vi "open_plotter.vi"(10 "Break":refnum<vi>) -> ()   [LabVIEW 2019]
panel:
  out "Output File Loaded?":bool
  in  "Load Simulation":bool
  in  "Close":bool
  out "# Lines Plot":i32
  in  "Parameters to Plot":string(tree)="_3"
  out "Output Files Path":path caption="selected path"
  in  "Open Button":bool
  in  "Clear Plot Selection":bool
  in  "Plot":bool
  # "Biogas Plotter"
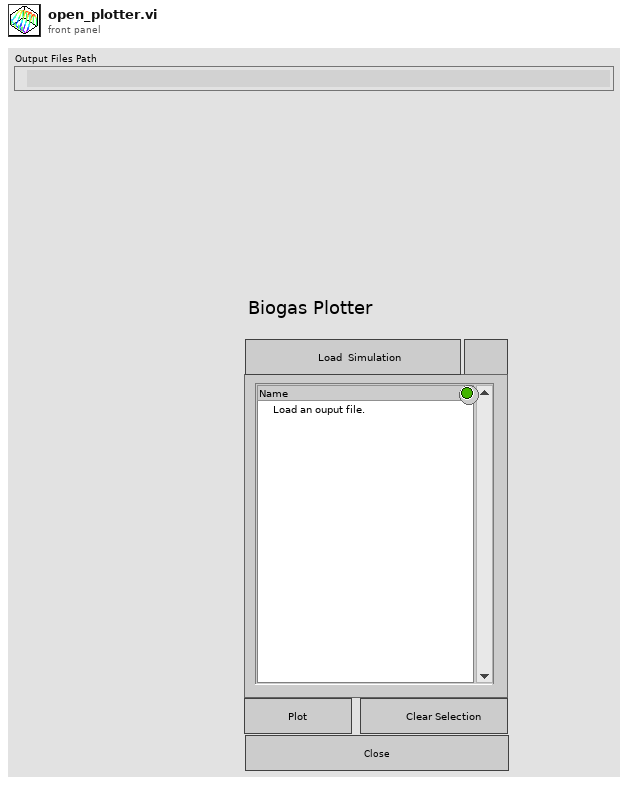
[diagram p1: front panel]
types:
  T1 = typedef "LVPoint32TypeDef.ctl" = cluster{"Horizontal":i32, "Vertical":i32}
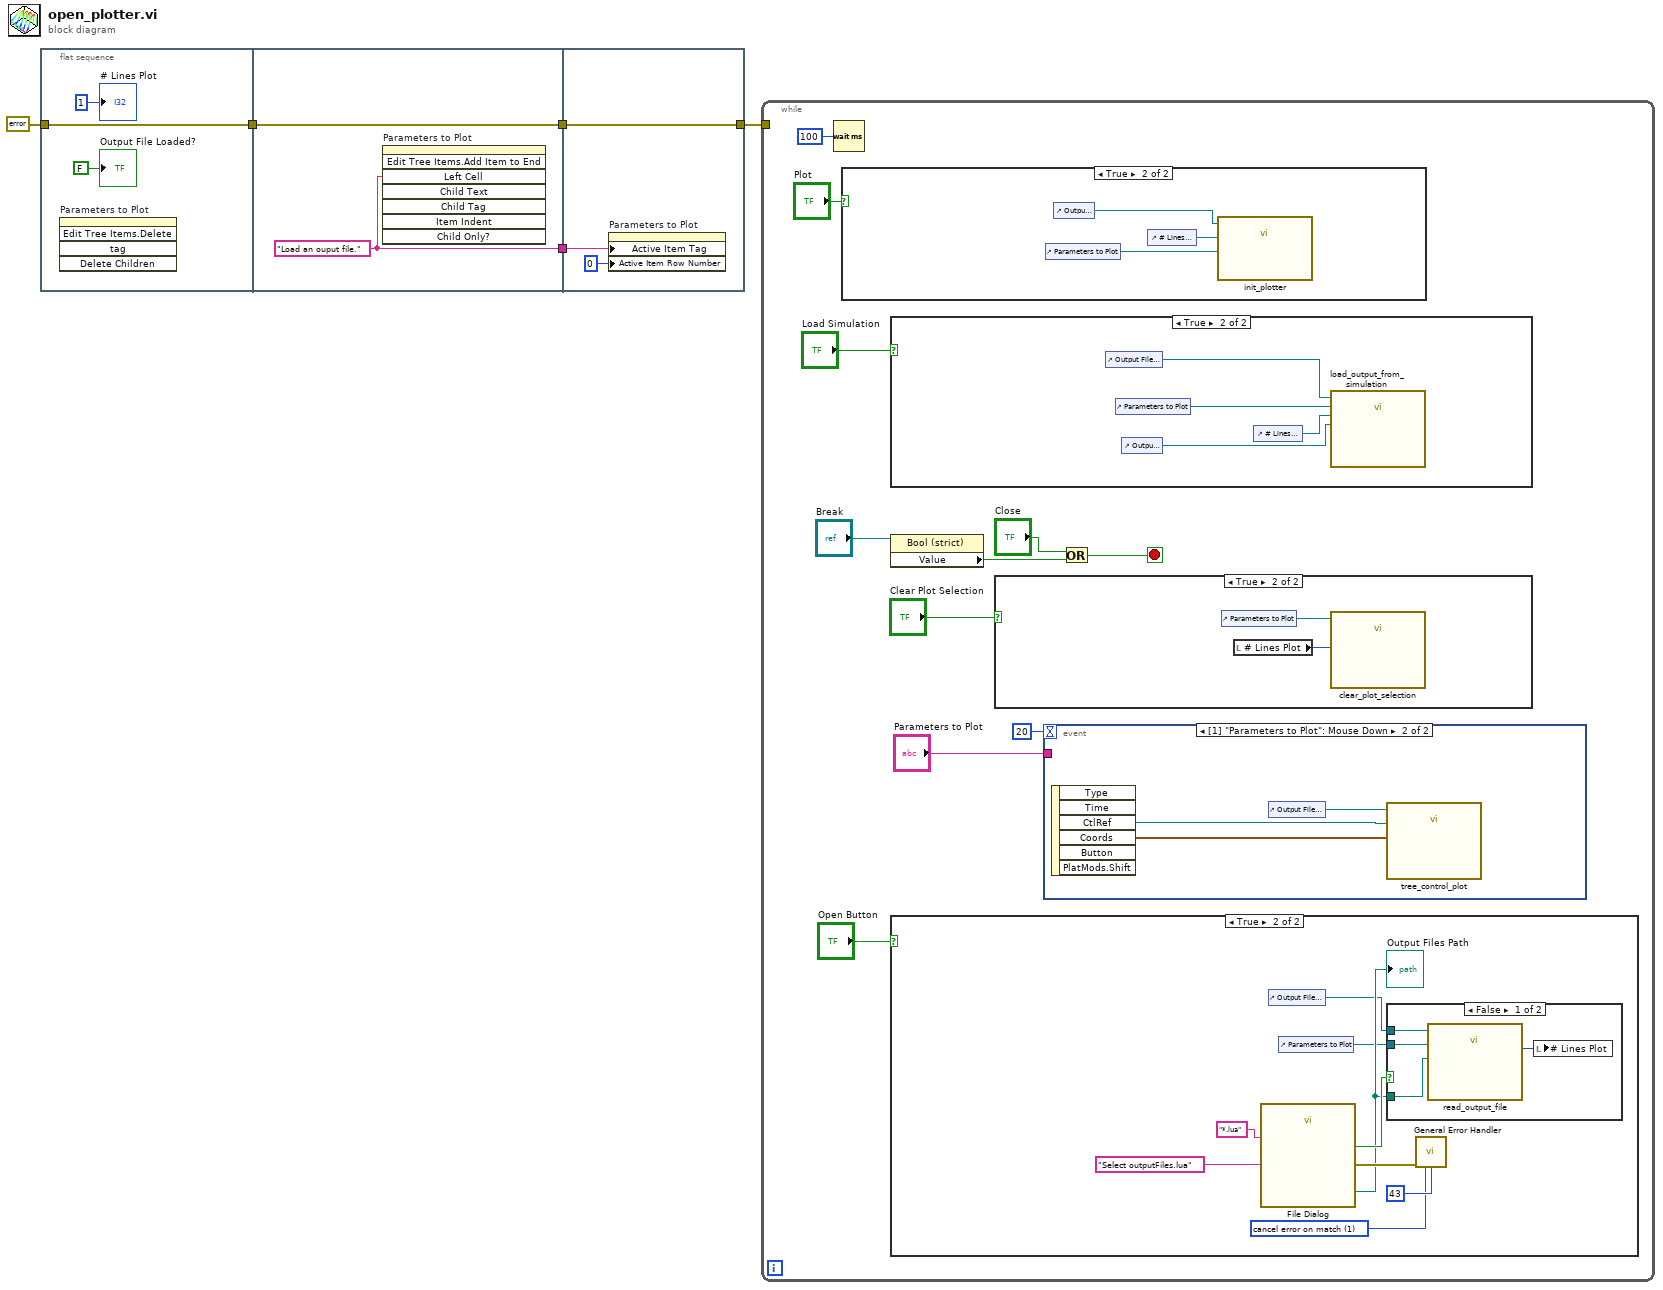
[diagram p0: block diagram]
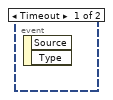
[diagram p6: hidden frame]
diagram:
  n1 = flat-sequence {
    tunnel: [w6] -> w3
    tunnel: errorcluster {"status"=FALSE, "code"=0, "source"=""} ("error constant") -> [w6]
    tunnel: [w10] -> w5
    tunnel: w3 -> [w9]
    tunnel: [w9] -> w2
    tunnel: w5 -> [w13]
    tunnel: w2 -> [w11]
    tunnel: [w11] -> w1
    frame #0 {
      n2 = invoke on="Parameters to Plot" class="Tree (strict)" method="Edit Tree Items.Delete"() -> ()  [unwired: 5 in, 5 out]
      "Output File Loaded?" <- FALSE ("Output File Loaded?")
      "# Lines Plot" <- 1 ("# Lines Plot")
    }
    frame #1 {
      w10 = "Load an ouput file." ("Left Cell String")
      n3 = invoke on="Parameters to Plot" class="Tree (strict)" method="Edit Tree Items.Add Item to End"("Left Cell"=w10) -> ()  [unwired: 7 in, 8 out]
    }
    frame #2 {
      n4 = property on="Parameters to Plot" class="Tree (strict)"("Active Item Tag"=w13, "Active Item Row Number"=0 ("Active Item:Row Number")) -> ()  [unwired: 2 in, 2 out]
    }
  }
  n5 = while {
    tunnel: w1 -> [_]
    stop <- w14 stop-if-true
    n6 = Wait (ms)(milliseconds to wait=u32 100) -> ()  [unwired: 1 out]
    n7 = case shown="True" "Plot" {
      frame False {
      }
      frame True {
        n8 = control-ref of="Parameters to Plot"() -> (w29:refnum<vi>)
        n9 = control-ref of="Output Files Path"() -> (w31:refnum<vi>)
        n10 = control-ref of="# Lines Plot"() -> (w30:refnum<vi>)
        n11 = call "init_plotter.vi"("Plot Tree"=w29, "#Lines Plot"=w30, "Output Files Path"=w31) -> ()  [unwired: 9 in]
      }
    }
    n12 = case shown="True" "Load Simulation" {
      frame False {
      }
      frame True {
        n13 = control-ref of="Output File Loaded?"() -> (w28:refnum<vi>)
        n14 = control-ref of="Parameters to Plot"() -> (w27:refnum<vi>)
        n15 = control-ref of="Output Files Path"() -> (w25:refnum<vi>)
        n16 = control-ref of="# Lines Plot"() -> (w26:refnum<vi>)
        n17 = call "load_output_from_simulation.vi"("Output Files Path"=w25, "# Lines Plot"=w26, "Parameters to Plot"=w27, "Output File Loaded?"=w28) -> ()  [unwired: 8 in]
      }
    }
    n18 = property class="Bool (strict)"(reference="Break") -> ("Value"=w15:bool)  [unwired: 1 in, 2 out]
    n19 = case shown="True" "Open Button" {
      frame False {
      }
      frame True {
        w38 = 1 items=["no exception", "cancel error on match", "set error on match"] ("[exception action] (none:0)")
        n20 = call "File Dialog"("prompt"="Select outputFiles.lua", "pattern (all files)"="*.lua") -> ("selected path"=w36:path, "cancelled"=w37:bool, "error out"=w40:errorcluster)  [unwired: 10 in, 1 out]
        "Output Files Path" <- w36
        n21 = control-ref of="Output File Loaded?"() -> (w34:refnum<vi>)
        n22 = control-ref of="Parameters to Plot"() -> (w35:refnum<vi>)
        n23 = case shown="False" w37 {
          tunnel: w36 -> [w44 _]
          tunnel: w35 -> [w43 _]
          tunnel: w34 -> [w42 _]
          frame False {
            n24 = call "read_output_file.vi"("TMP Filepath"=w44, "Plot Tree"=w43, "Output File Loaded?"=w42) -> ("# Lines Plot"=w41:i32)  [unwired: 8 in]
            n25 = local write "# Lines Plot"(w41) -> ()
          }
          frame True {
          }
        }
        n26 = call <vilib>:"General Error Handler.vi"("error in (no error)"=w40, "[exception action] (none:0)"=w38, "[exception code]"=43) -> ()  [unwired: 8 in, 5 out]
      }
    }
    n27 = case shown="True" "Clear Plot Selection" {
      frame False {
      }
      frame True {
        n28 = control-ref of="Parameters to Plot"() -> (w48:refnum<vi>)
        n29 = local read "# Lines Plot"() -> (w49:i32)
        n30 = call "clear_plot_selection.vi"("# Lines Plot"=w49, "Plot Tree"=w48) -> ()  [unwired: 10 in]
      }
    }
    n31 = event shown="[1] \"Parameters to Plot\": Mouse Down" {
      selector: _ -> [_ _]
      dyn-events: _ -> [_ _]
      timeout: 20 -> [_ _]
      tunnel: "Parameters to Plot" -> [_ _]
      event Timeout {
        n32 = event-data() -> ()  [unwired: 1 in, 2 out]
      }
      event "Parameters to Plot": Mouse Down {
        n33 = event-data() -> ("CtlRef"=w47:refnum<vi>, "Coords"=w46:T1)  [unwired: 1 in, 4 out]
        n34 = control-ref of="Output File Loaded?"() -> (w45:refnum<vi>)
        n35 = call "tree_control_plot.vi"("Point"=w46, "Plot Tree"=w47, "Output File Loaded?"=w45) -> ()  [unwired: 9 in]
      }
    }
    n36 = Or(x="Close", y=w15) -> (x .or. y?=w14:bool)
  }
